vi "ResultReadOut.vi"(11 "Str_Result?":string="1,-1.7619E-13,2,2,2,-9.2453E-14,2,2,3,-1.8474E-13,2,2,4,-2.2100E-13,2,2") -> (0 "MeasuredValue4":dbl format="%#_6e", 1 "MeasuredValue3":dbl format="%#_6e", 2 "MeasuredValue2":dbl format="%#_6e", 3 "MeassuredValue1":dbl format="%#_6e")   [LabVIEW 2016]
panel:
  out "ch1":i32
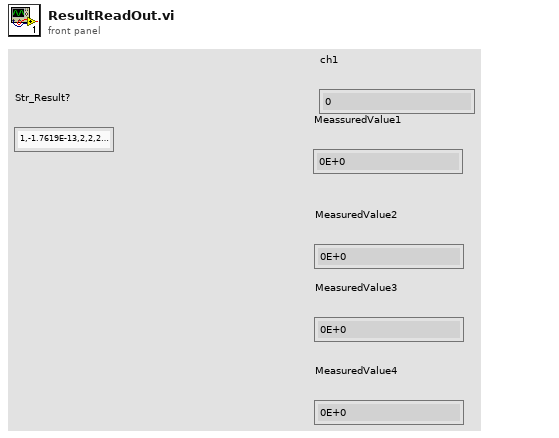
[diagram p1: front panel]
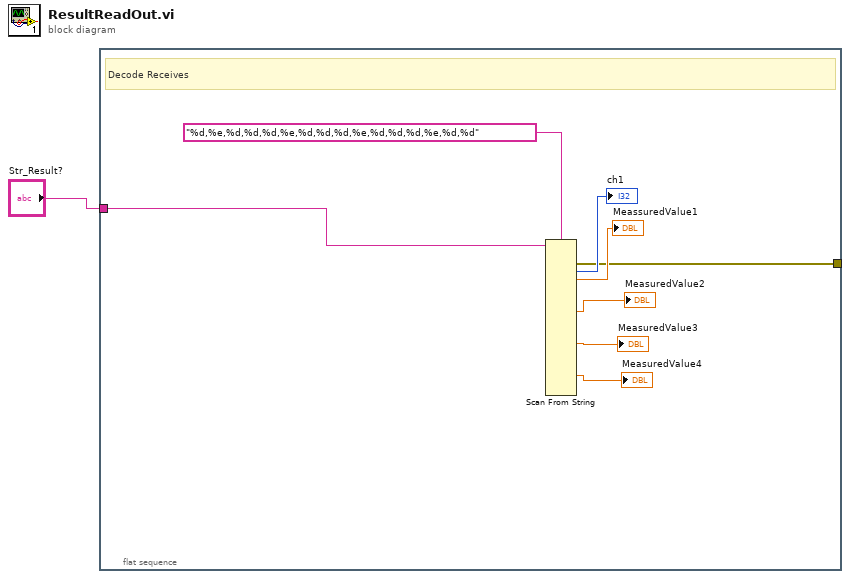
[diagram p0: block diagram]
diagram:
  n1 = flat-sequence {
    tunnel: "Str_Result?" -> [w6]
    tunnel: [w2] -> _
    frame #0 {
      # "Decode Receives"
      n2 = Scan From String(format string="%d,%e,%d,%d,%d,%e,%d,%d,%d,%e,%d,%d,%d,%e,%d,%d", input string=w6) -> (error out=w2:errorcluster, output 1=→"ch1":i32, output 2=→"MeassuredValue1":dbl, output 6=→"MeasuredValue2":dbl, output 10=→"MeasuredValue3":dbl, output 14=→"MeasuredValue4":dbl)  [unwired: 29 in, 2 out]
    }
  }
